vi "Registrar-Usuarios.vi"() -> ()   [LabVIEW 2024]
uses:
  <vilib>/Utility/file.llb/Read Delimited Spreadsheet (string).vi
  <vilib>/Utility/file.llb/Write Delimited Spreadsheet (string).vi
panel:
  out "Path":path=path "C:/Users/willi/GITHUB/TG/OBJ 2 - RECOLECCION DE DATOS/registro-usuarios.csv"
  out "Usserr":i32
  out "NextUser":i32
  in  "Registrar Usuario":T1 {"Edad" format="%#_13g"}
  in  "registrButt":bool
  in  "stop":bool
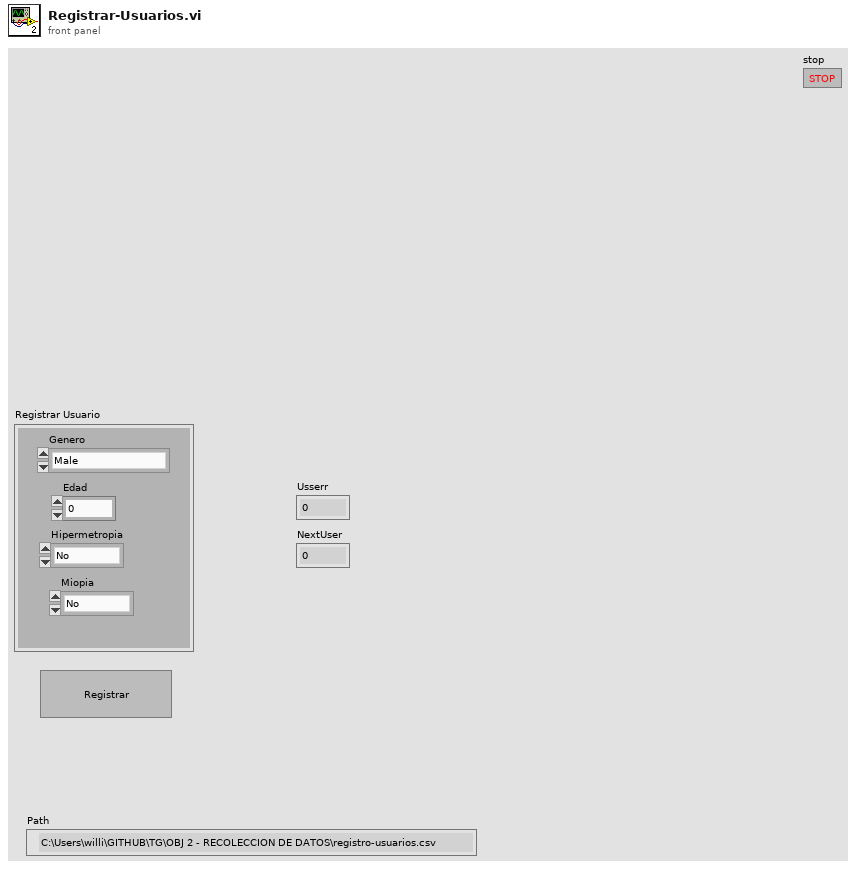
[diagram p1: front panel]
types:
  T1 = cluster{"Genero":enum16{"Male", "Female"}, "Edad":dbl, "Hipermetropia":enum16{"No", "Si"}, "Miopia":enum16{"No", "Si"}}
  T2 = cluster{"Usuario":i32, "Genero":enum16{"Male", "Female"}, "Edad":dbl, "Hipermetropia":enum16{"No", "Si"}, "Miopia":enum16{"No", "Si"}}
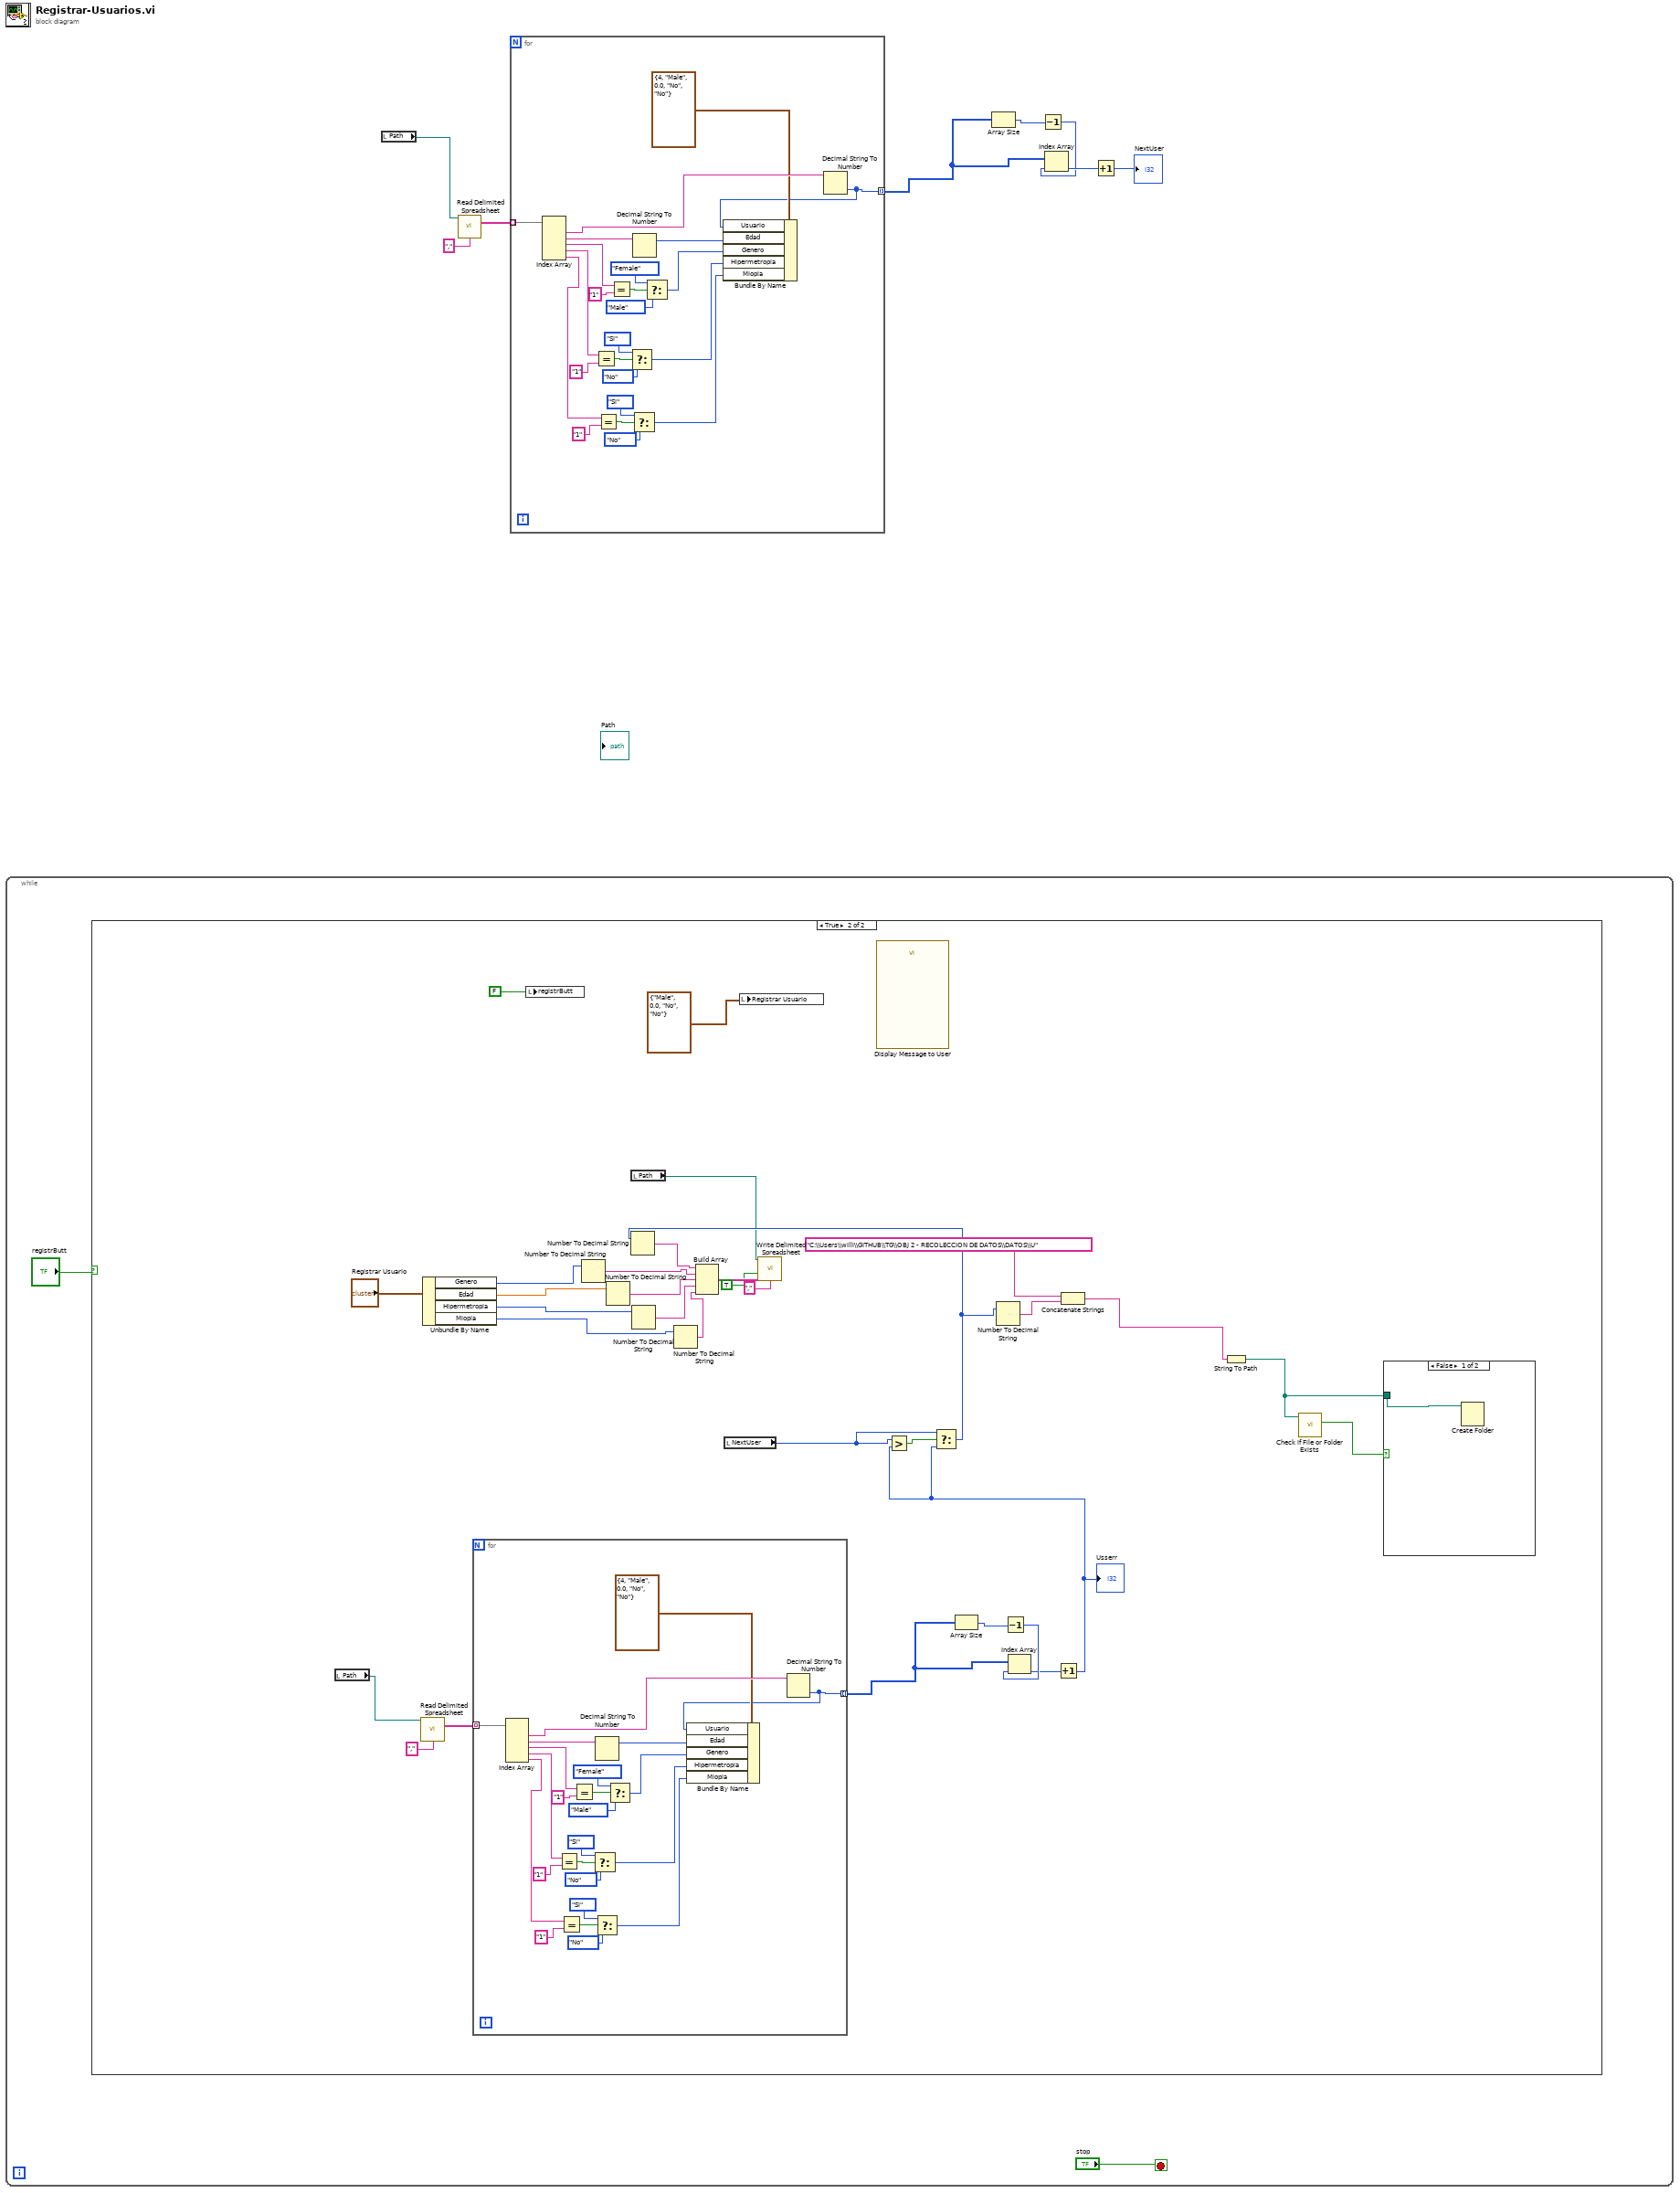
[diagram p0: block diagram]
diagram:
  n1 = while {
    stop <- "stop" stop-if-true
    n2 = case shown="True" "registrButt" {
      frame False {
      }
      frame True {
        n3 = local read "Path"() -> (w15:path)
        n4 = call-poly <vilib>:"Read Delimited Spreadsheet.vi"("file path (dialog if empty)"=w15, "delimiter (\\t)"="," ("delimiter (\\t)")) -> ("all rows"=w27:string[][])  [unwired: 8 in, 5 out]
        n5 = Unbundle By Name("Registrar Usuario") -> ("Genero"=w32:enum16{"Male", "Female"}, "Edad"=w31:dbl, "Hipermetropia"=w30:enum16{"No", "Si"}, "Miopia"=w29:enum16{"No", "Si"})
        n6 = for {
          tunnel: w27 -> [w67] mode=indexing
          tunnel: [w44] -> w26 mode=indexing
          n7 = Index Array(array=w67) -> (element #1=w48:string, element #2=w46:string, element #3=w65:string, element #4=w56:string, element #5=w50:string)  [unwired: 5 in]
          n8 = Equal?(x=w56, y="1") -> (x = y?=w59:bool)
          n9 = Equal?(x=w50, y="1") -> (x = y?=w53:bool)
          n10 = Equal?(x=w65, y="1") -> (x = y?=w64:bool)
          n11 = Select(t=enum16{"No", "Si"}."Si" ("Hipermetropia"), s=w59, f=enum16{"No", "Si"}."No" ("Hipermetropia")) -> (s? t:f=w55:enum16{"No", "Si"})
          n12 = Decimal String To Number(string=w46) -> (offset past number=w45:i32)  [unwired: 2 in, 1 out]
          n13 = Select(t=enum16{"No", "Si"}."Si" ("Hipermetropia"), s=w53, f=enum16{"No", "Si"}."No" ("Hipermetropia")) -> (s? t:f=w49:enum16{"No", "Si"})
          n14 = Select(t=enum16{"Male", "Female"}."Female" ("Genero"), s=w64, f=enum16{"Male", "Female"}."Male" ("Genero")) -> (s? t:f=w61:enum16{"Male", "Female"})
          n15 = Decimal String To Number(string=w48) -> (number=w44:i32)  [unwired: 2 in, 1 out]
          n16 = Bundle By Name(cluster=T2 {"Usuario"=4, "Genero"=enum."Male", "Edad"=0.0, "Hipermetropia"=enum."No", "Miopia"=enum."No"} ("Registrar Usuario"), "Usuario"=w44, "Edad"=w45, "Genero"=w61, "Hipermetropia"=w55, "Miopia"=w49) -> ()  [unwired: 1 out]
        }
        n17 = local write "registrButt"(FALSE) -> ()
        n18 = Number To Decimal String(number=w32) -> (decimal integer string=w33:string)  [unwired: 1 in]
        n19 = Number To Decimal String(number=w31) -> (decimal integer string=w36:string)  [unwired: 1 in]
        n20 = local read "Path"() -> (w14:path)
        n21 = Number To Decimal String(number=w30) -> (decimal integer string=w37:string)  [unwired: 1 in]
        n22 = Number To Decimal String(number=w29) -> (decimal integer string=w38:string)  [unwired: 1 in]
        n23 = local read "NextUser"() -> (w20:i32)
        n24 = local write "Registrar Usuario"(T1 {"Genero"=enum."Male", "Edad"=0.0, "Hipermetropia"=enum."No", "Miopia"=enum."No"} ("Registrar Usuario")) -> ()
        n25 = call "Display Message to User"() -> ()  [unwired: 10 in, 2 out]
        n26 = Array Size(array=w26) -> (size(s)=w25:i32)
        n27 = Decrement(x=w25) -> (x-1=w24:i32)
        n28 = Index Array(array=w26, index=w24) -> (element=w23:i32)
        n29 = Increment(x=w23) -> (x+1=w19:i32)
        "Usserr" <- w19
        n30 = Greater?(x=w20, y=w19) -> (0:w21:bool)
        n31 = Select(t=w20, s=w21, f=w19) -> (s? t:f=w18:i32)
        n32 = Number To Decimal String(number=w18) -> (decimal integer string=w28:string)  [unwired: 1 in]
        n33 = Build Array(w28, w33, w36, w37, w38) -> (w41:string[])
        n34 = call-poly <vilib>:"Write Delimited Spreadsheet.vi"("file path (dialog if empty)"=w14, "1D data"=w41, "append to file? (new file:F)"=TRUE, "delimiter (\\t)"="," ("delimiter (\\t)")) -> ()  [unwired: 10 in, 2 out]
        n35 = Number To Decimal String(number=w18) -> (decimal integer string=w17:string)  [unwired: 1 in]
        n36 = Concatenate Strings("C:\\Users\\willi\\GITHUB\\TG\\OBJ 2 - RECOLECCION DE DATOS\\DATOS\\U" ("string"), w17) -> (w13:string)
        n37 = String To Path(string=w13) -> (path=w11:path)
        n38 = call <vilib>:"Check if File or Folder Exists.vi"("path"=w11) -> ("file or folder exists?"=w12:bool)  [unwired: 8 in, 2 out]
        n39 = case shown="False" w12 {
          tunnel: w11 -> [w43 _]
          frame False {
            n40 = Create Folder(path (use dialog)=w43) -> ()  [unwired: 2 in, 3 out]
          }
          frame True {
          }
        }
      }
    }
  }
  n41 = local read "Path"() -> (w2:path)
  n42 = call-poly <vilib>:"Read Delimited Spreadsheet.vi"("file path (dialog if empty)"=w2, "delimiter (\\t)"="," ("delimiter (\\t)")) -> ("all rows"=w4:string[][])  [unwired: 8 in, 5 out]
  n43 = for {
    tunnel: w4 -> [w91] mode=indexing
    tunnel: [w68] -> w1 mode=indexing
    n44 = Index Array(array=w91) -> (element #1=w72:string, element #2=w70:string, element #3=w89:string, element #4=w80:string, element #5=w74:string)  [unwired: 5 in]
    n45 = Equal?(x=w80, y="1") -> (x = y?=w83:bool)
    n46 = Equal?(x=w74, y="1") -> (x = y?=w77:bool)
    n47 = Equal?(x=w89, y="1") -> (x = y?=w88:bool)
    n48 = Select(t=enum16{"No", "Si"}."Si" ("Hipermetropia"), s=w83, f=enum16{"No", "Si"}."No" ("Hipermetropia")) -> (s? t:f=w79:enum16{"No", "Si"})
    n49 = Decimal String To Number(string=w70) -> (offset past number=w69:i32)  [unwired: 2 in, 1 out]
    n50 = Select(t=enum16{"No", "Si"}."Si" ("Hipermetropia"), s=w77, f=enum16{"No", "Si"}."No" ("Hipermetropia")) -> (s? t:f=w73:enum16{"No", "Si"})
    n51 = Select(t=enum16{"Male", "Female"}."Female" ("Genero"), s=w88, f=enum16{"Male", "Female"}."Male" ("Genero")) -> (s? t:f=w85:enum16{"Male", "Female"})
    n52 = Decimal String To Number(string=w72) -> (number=w68:i32)  [unwired: 2 in, 1 out]
    n53 = Bundle By Name(cluster=T2 {"Usuario"=4, "Genero"=enum."Male", "Edad"=0.0, "Hipermetropia"=enum."No", "Miopia"=enum."No"} ("Registrar Usuario"), "Usuario"=w68, "Edad"=w69, "Genero"=w85, "Hipermetropia"=w79, "Miopia"=w73) -> ()  [unwired: 1 out]
  }
  n54 = Array Size(array=w1) -> (size(s)=w5:i32)
  n55 = Decrement(x=w5) -> (x-1=w6:i32)
  n56 = Index Array(array=w1, index=w6) -> (element=w7:i32)
  n57 = Increment(x=w7) -> (x+1=→"NextUser":i32)
